vi "FVer (Read).vi"(6 "ISOBUS address":T2=-1 caption="ISOBUS address (-1)", 8 "error in":errorcluster, 11 "Mercury Reference In":T3) -> (0 "error out":errorcluster, 2 "Firmware Version":string, 3 "Mercury Reference Out":T3, 4 "Valid?":T1)   [LabVIEW 2019, in "Mercury iXX.lvlib" / "System.lvlib"]
doc: "Returns the firmware version of the selected device."
uses:
  System.lvlib
  Controls/Mercury Reference.ctl
  Controls/Comms Transport Layer.ctl
  Private/Controls/Query Dynamic Reference.ctl
  Controls/ISOBus Address.ctl
  Controls/Is Valid LED.ctl
  Private/Controls/Command Verbs.ctl
  Mercury iXX.lvlib
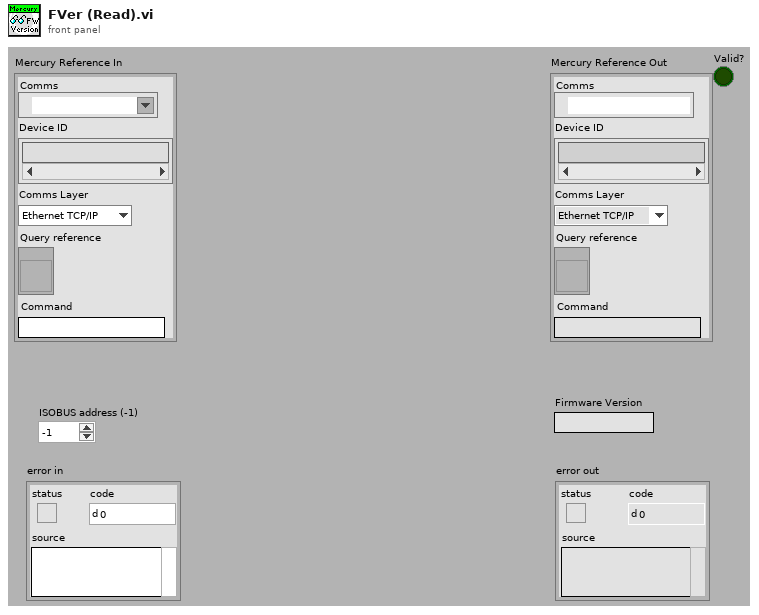
[diagram p1: front panel]
types:
  T1 = typedef "Mercury iXX.lvlib/Is Valid LED.ctl" = bool
  T2 = typedef "Mercury iXX.lvlib/ISOBus Address.ctl" = i32
  T3 = typedef "Mercury iXX.lvlib/Mercury Reference.ctl" = cluster{"Comms":refnum<visa-resource-name>, "Device ID":string[], "Comms Layer":T4, "Command":string, "Query reference":T5}
  T4 = typedef "Mercury iXX.lvlib/Comms Transport Layer.ctl" = enum16{"Ethernet TCP/IP", "USB", "ISOBus - RS-232", "GPIB"}
  T5 = typedef "Mercury iXX.lvlib/Query Dynamic Reference.ctl" = refnum<vi>
  T6 = typedef "Mercury iXX.lvlib/Command Verbs.ctl" = string
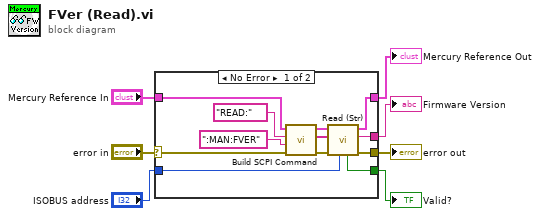
[diagram p0: block diagram]
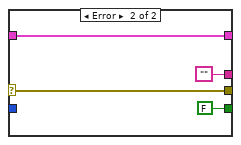
[diagram p2: hidden frame]
diagram:
  n1 = case shown="No Error" "error in" {
    selector: "error in" -> [w9 w22]
    tunnel: "Mercury Reference In" -> [w12 w23]
    tunnel: [w18 w23] -> w6
    tunnel: [w17 w22] -> w5
    tunnel: "ISOBUS address" -> [w15 _]
    tunnel: [w14 ""] -> w2
    tunnel: [w16 FALSE ("Valid?")] -> w1
    frame No Error {
      n2 = call "Build SCPI Command.vi"("error in"=w9, "Noun(s)"=":MAN:FVER", "Verb"=T6 "READ:", "Mercury Reference In"=w12) -> ("error out"=w8:errorcluster, "SCPI Message(s)"=w13:string[], "Mercury Reference Out"=w11:T3)  [unwired: 5 out]
      n3 = call "Read (Str).vi"("ISOBUS address"=w15, "error in"=w8, "SCPI Message(s)"=w13, "Mercury Reference In"=w11) -> ("error out"=w17:errorcluster, "Response"=w14:string, "Mercury Reference Out"=w18:T3, "Valid?"=w16:T1)  [unwired: 4 out]
    }
    frame Error {
    }
  }
  "Mercury Reference Out" <- w6
  "error out" <- w5
  "Firmware Version" <- w2
  "Valid?" <- w1
